vi "IT8800-Request.vi"(6 "Response?":bool=TRUE, 8 "error in":errorcluster, 9 "byte count":u32, 10 "Command":string, 11 "IT8800 Setting In In":T1={"VISA Resource Name"="", "Baud Rate"=19200, "Stop Bits"=20, "Wait For Read(ms)"=0, "Interface Type"=enum."VXI", "Limits"=[]} {"Stop Bits" items=["1.0"=10, "2.0"=20]; "Baud Rate" items=["2400"=2400, "4800"=4800, "9600"=9600, "19200"=19200]}) -> (0 "error out":errorcluster, 2 "Response":string, 3 "IT8800 Setting In Out":T1={"VISA Resource Name"="", "Baud Rate"=19200, "Stop Bits"=20, "Wait For Read(ms)"=0, "Interface Type"=enum."VXI", "Limits"=[]} {"Stop Bits" items=["1.0"=10, "2.0"=20]; "Baud Rate" items=["2400"=2400, "4800"=4800, "9600"=9600, "19200"=19200]})   [LabVIEW 2018]
uses:
  Data Def/IT8800-Setting.ctl
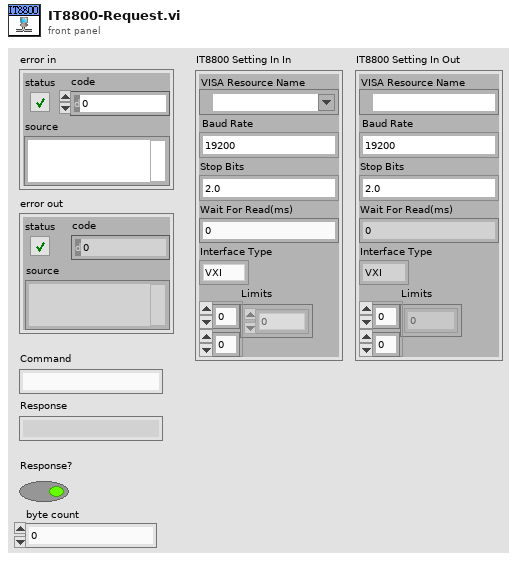
[diagram p1: front panel]
types:
  T1 = typedef "IT8800-Setting.ctl" = cluster{"VISA Resource Name":refnum<visa-resource-name>, "Baud Rate":u32, "Stop Bits":u16, "Wait For Read(ms)":u32, "Interface Type":enum16{"Unknow", "GPIB", "VXI", "GPIB-VXI", "Serial", "PXI", "TCPIP", "USB", "FireWire"}, "Limits":dbl[][]}
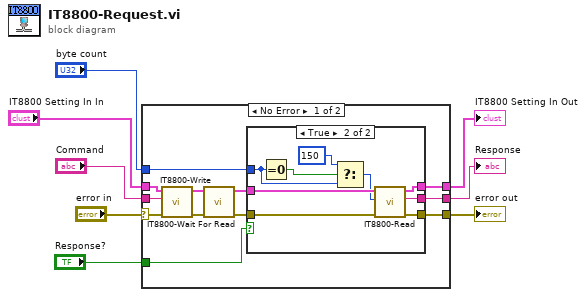
[diagram p0: block diagram]
diagram:
  n1 = case shown="No Error" "error in" {
    selector: "error in" -> [w18 w33]
    tunnel: [w20 w33] -> w8
    tunnel: "Response?" -> [w13 _]
    tunnel: "Command" -> [w17 _]
    tunnel: [w15 _] -> w5
    tunnel: "IT8800 Setting In In" -> [w16 w32]
    tunnel: "byte count" -> [w19 _]
    tunnel: [w14 w32] -> w1
    frame No Error {
      n2 = call "IT8800-Write.vi"("error in"=w18, "Command"=w17, "IT8800 Setting In In"=w16) -> ("error out"=w12:errorcluster, "IT8800 Setting In Out"=w10:T1)  [unwired: 7 in]
      n3 = call "IT8800-Wait For Read.vi"("error in"=w12, "IT8800 Setting In In"=w10) -> ("error out"=w11:errorcluster, "IT8800 Setting In Out"=w9:T1)  [unwired: 8 in]
      n4 = case shown="True" w13 {
        tunnel: [w22 w31] -> w20
        tunnel: w19 -> [_ w30]
        tunnel: w9 -> [w21 w29]
        tunnel: [_ w28] -> w15
        tunnel: [w21 w27] -> w14
        tunnel: w11 -> [w22 w24]
        frame False {
        }
        frame True {
          n5 = Equal To 0?(x=w30) -> (x = 0?=w26:bool)
          n6 = Select(t=u32 150 ("byte count"), s=w26, f=w30) -> (s? t:f=w23:u32)
          n7 = call "IT8800-Read.vi"("error in"=w24, "byte count"=w23, "IT8800 Setting In In"=w29) -> ("error out"=w31:errorcluster, "Response"=w28:string, "IT8800 Setting In Out"=w27:T1)  [unwired: 6 in]
        }
      }
    }
    frame Error {
    }
  }
  "error out" <- w8
  "IT8800 Setting In Out" <- w1
  "Response" <- w5
